vi "Menue.vi"() -> ()   [LabVIEW 2012]
panel:
  in  "start vi2":bool
  in  "start vi1":bool
  in  "start vi3":bool
  in  "stop":bool
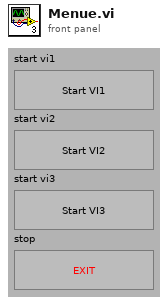
[diagram p1: front panel]
types:
  T1 = enum32{"Invalid", "Standard", "Closed", "Hidden", "Minimized", "Maximized"}
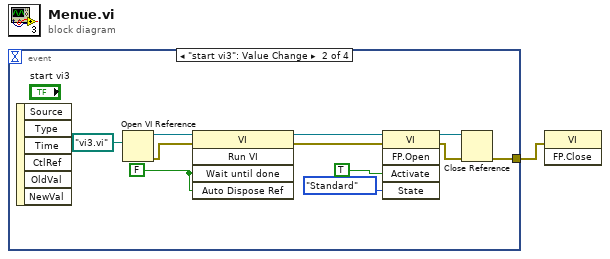
[diagram p0: block diagram]
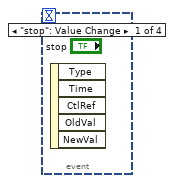
[diagram p2: hidden frame]
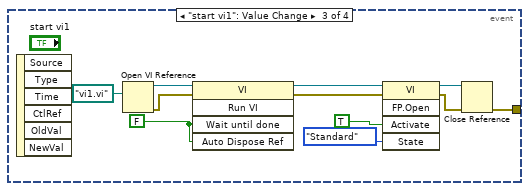
[diagram p3: hidden frame]
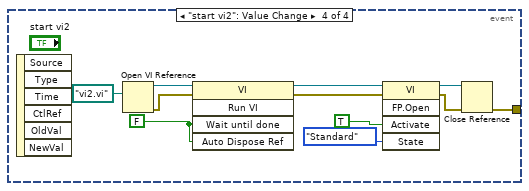
[diagram p4: hidden frame]
diagram:
  n1 = event shown="[1] \"start vi3\": Value Change" {
    selector: _ -> [_ _ _ _]
    dyn-events: _ -> [_ _ _ _]
    timeout: _ -> [_ _ _ _]
    tunnel: [_ w2 w13 w24] -> w1
    event "stop": Value Change {
      n2 = event-data() -> ()  [unwired: 6 out]
    }
    event "start vi3": Value Change {
      w10 = FALSE ("Wait Until Done")
      n3 = event-data() -> ()  [unwired: 7 out]
      n4 = Open VI Reference(vi path=path "vi3.vi") -> (vi reference=w11:refnum<vi>, error out=w9:errorcluster)  [unwired: 1 in, 4 out]
      n5 = invoke class="VI" method="Run VI"(reference=w11, error in=w9, "Wait until done"=w10, "Auto Dispose Ref"=w10) -> (reference out=w8:refnum<vi>, error out=w7:errorcluster)  [unwired: 1 in, 3 out]
      n6 = invoke class="VI" method="FP.Open"(reference=w8, error in=w7, "Activate"=TRUE ("Activate?"), "State"=T1."Standard") -> (reference out=w6:refnum<vi>, error out=w5:errorcluster)  [unwired: 1 in, 3 out]
      n7 = Close Reference(reference=w6, error in (no error)=w5) -> (error out=w2:errorcluster)
    }
    event "start vi1": Value Change {
      w21 = FALSE ("Wait Until Done")
      n8 = event-data() -> ()  [unwired: 7 out]
      n9 = Open VI Reference(vi path=path "vi1.vi") -> (vi reference=w22:refnum<vi>, error out=w20:errorcluster)  [unwired: 1 in, 4 out]
      n10 = invoke class="VI" method="Run VI"(reference=w22, error in=w20, "Wait until done"=w21, "Auto Dispose Ref"=w21) -> (reference out=w19:refnum<vi>, error out=w18:errorcluster)  [unwired: 1 in, 3 out]
      n11 = invoke class="VI" method="FP.Open"(reference=w19, error in=w18, "Activate"=TRUE ("Activate?"), "State"=T1."Standard") -> (reference out=w17:refnum<vi>, error out=w16:errorcluster)  [unwired: 1 in, 3 out]
      n12 = Close Reference(reference=w17, error in (no error)=w16) -> (error out=w13:errorcluster)
    }
    event "start vi2": Value Change {
      w32 = FALSE ("Wait Until Done")
      n13 = event-data() -> ()  [unwired: 7 out]
      n14 = Open VI Reference(vi path=path "vi2.vi") -> (vi reference=w33:refnum<vi>, error out=w31:errorcluster)  [unwired: 1 in, 4 out]
      n15 = invoke class="VI" method="Run VI"(reference=w33, error in=w31, "Wait until done"=w32, "Auto Dispose Ref"=w32) -> (reference out=w30:refnum<vi>, error out=w29:errorcluster)  [unwired: 1 in, 3 out]
      n16 = invoke class="VI" method="FP.Open"(reference=w30, error in=w29, "Activate"=TRUE ("Activate?"), "State"=T1."Standard") -> (reference out=w28:refnum<vi>, error out=w27:errorcluster)  [unwired: 1 in, 3 out]
      n17 = Close Reference(reference=w28, error in (no error)=w27) -> (error out=w24:errorcluster)
    }
  }
  n18 = invoke class="VI" method="FP.Close"(error in=w1) -> ()  [unwired: 2 in, 3 out]
